vi "State_Machine.vi"(8 "error in (no error)":errorcluster caption="entrée d'erreur (pas d'erreur)", 11 "Enable_DIO en entrée":refnum<class "Disable_DIO.lvclass">) -> (0 "error out":errorcluster caption="sortie d'erreur", 2 "Json_String":string, 3 "Enable_DIO en sortie":refnum<class "Disable_DIO.lvclass">)   [LabVIEW 2020, in "Library Test.lvlib" / "Disable_DIO.lvclass"]
uses:
  Disable_DIO.lvclass
  C:/Users/ngarcin/OneDrive - Altyor/Standard TB/Class/Test/Test (Default)/Test (Default).lvclass
  JSON API/Variant JSON/Variant to JSON.vi
  JSON API/JSON Value/Get Item by name array.vi
  Instrument/Instrument (Default)/Class Instrument (Default).lvclass
  JSON API/JSON Value/JSON Value.lvclass
  Disable_DIO.lvclass/Disable_DIO.ctl
  JSON API/Get Polymorphic/JSON GetSet.lvlib
  JSON API/Variant JSON/Variant JSON.lvlib
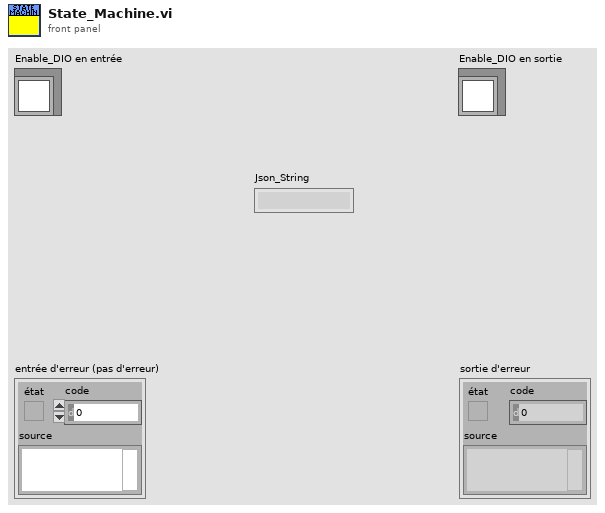
[diagram p1: front panel]
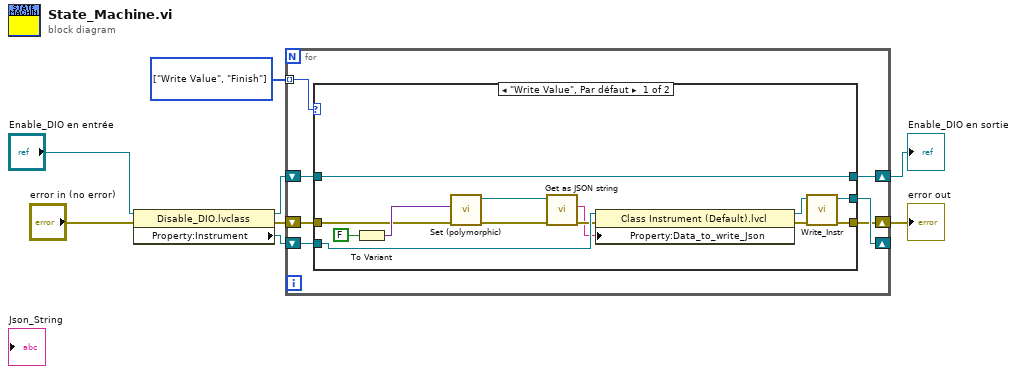
[diagram p0: block diagram]
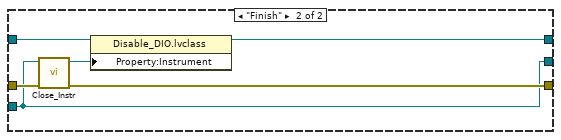
[diagram p2: hidden frame]
diagram:
  w7 = enum16{"Init", "Write Value", "Finish"}[] [enum."Write Value", enum."Finish"] items=["Init", "Write Value", "Finish"]
  n1 = property class="Disable_DIO.lvclass"(reference="Enable_DIO en entrée", error in="error in (no error)") -> (reference out=w5:refnum<class "Disable_DIO.lvclass">, error out=w1:errorcluster, "Property:Instrument"=w6:refnum<class "Class Instrument (Default).lvclass">)
  n2 = for {
    tunnel: w7 -> [w15] mode=indexing
    shift-right: [w13] -> _
    shift-left: w6 -> [w14]
    shift-right: [w11] -> w3
    shift-left: w5 -> [w12]
    shift-right: [w9] -> w4
    shift-left: w1 -> [w10]
    n3 = case shown="\"Write Value\", Par défaut" w15 {
      tunnel: w14 -> [w25 w30]
      tunnel: [w26 w30] -> w13
      tunnel: w12 -> [w28 w34]
      tunnel: [w28 w33] -> w11
      tunnel: w10 -> [w19 w32]
      tunnel: [w27 w31] -> w9
      frame "Write Value", Default {
        n4 = To Variant(anything=FALSE) -> (Variant=w22:variant)
        n5 = call-poly "Set (polymorphic).vi"("error in (no error)"=w19, "Variant"=w22) -> ("error out"=w20:errorcluster, "JSON Value out"=w21:refnum<class "JSON Value.lvclass">)  [unwired: 8 in]
        n6 = call "Get as JSON string.vi"("error in (no error)"=w20, "JSON Value in"=w21) -> ("error out"=w18:errorcluster, "<JSON>"=w16:string)  [unwired: 8 in]
        n7 = property class="Class Instrument (Default).lvcl"(reference=w25, error in=w18, "Property:Data_to_write_Json"=w16) -> (reference out=w24:refnum<class "Class Instrument (Default).lvclass">, error out=w23:errorcluster)
        n8 = call-dynamic "Write_Instr.vi"("error in (no error)"=w23, "Class Multimeter (Default) en entrée"=w24) -> ("error out"=w27:errorcluster, "Class Multimeter (Default) en sortie"=w26:refnum<class "Class Instrument (Default).lvclass">)  [unwired: 8 in]
      }
      frame "Finish" {
        n9 = call-dynamic "Close_Instr.vi"("error in (no error)"=w32, "Class Instrument (Default) en entrée"=w30) -> ("error out"=w31:errorcluster, "Class Instrument (Default) en sortie"=w29:refnum<class "Class Instrument (Default).lvclass">)  [unwired: 8 in]
        n10 = property class="Disable_DIO.lvclass"(reference=w34, "Property:Instrument"=w29) -> (reference out=w33:refnum<class "Disable_DIO.lvclass">)  [unwired: 1 in, 1 out]
      }
    }
  }
  "error out" <- w4
  "Enable_DIO en sortie" <- w3
